vi "VISA GPIB Test.vi"() -> ()   [LabVIEW 2015]
panel:
  out "read buffer":string
  in  "write buffer":string
  # "++mode [0]|[1] to change between controller and device\n++mode to read back current mode\n\n++addr to read back the currently set address\n++addr [#] to set the addr of the device to talk to/address of the emulated device\n\nOnce mode and addr are set correctly\nOPEN 100 open relay 100\nCLOSE 100 close relay 100"
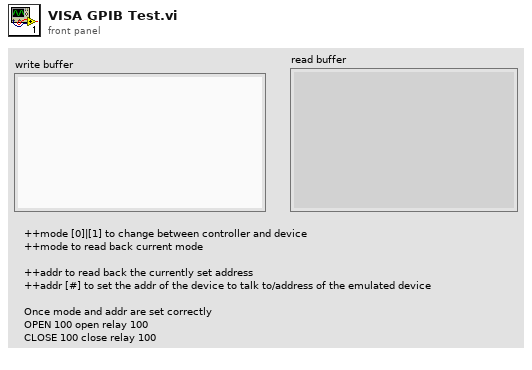
[diagram p1: front panel]
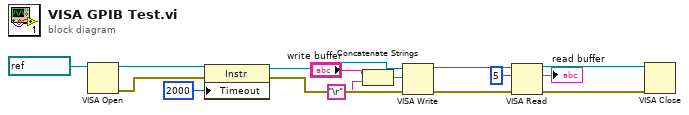
[diagram p0: block diagram]
diagram:
  n1 = VISA Open(VISA resource name=refnum<visa-resource-name> "COM4") -> (VISA resource name=w8:refnum<visa-resource-name>, error out=w7:errorcluster)  [unwired: 4 in]
  n2 = property class="Instr"(reference=w8, error in=w7, "Timeout"=u32 2000 ("General Settings:Timeout Value")) -> (reference out=w6:refnum<visa-resource-name>, error out=w5:errorcluster)
  n3 = Concatenate Strings("write buffer", "\r") -> (w3:string)
  n4 = VISA Write(VISA resource name=w6, write buffer=w3, error in (no error)=w5) -> (VISA resource name out=w14:refnum<visa-resource-name>, error out=w13:errorcluster)  [unwired: 1 out]
  n5 = VISA Read(VISA resource name=w14, byte count=u32 5, error in (no error)=w13) -> (VISA resource name out=w11:refnum<visa-resource-name>, read buffer=→"read buffer":string, error out=w10:errorcluster)  [unwired: 1 out]
  n6 = VISA Close(VISA resource name=w11, error in (no error)=w10) -> ()  [unwired: 1 out]
